vi "DoCreateError.vi"(5 "MergeErrors":bool, 6 "AdditionalText":string, 7 "Data":variant, 8 "ErrorIn":errorcluster caption="Error In", 9 "Text":string, 10 "ErrorCode":i32, 11 "ObjectIn":refnum<class "ErrorCreationJSON.lvclass"> caption="Object In") -> (0 "ErrorOut":errorcluster caption="Error Out", 3 "ObjectOut":refnum<class "ErrorCreationJSON.lvclass"> caption="Object Out")   [LabVIEW 2021, in "ErrorCreationJSON.lvclass"]
uses:
  ErrorCreationJSON.lvclass
  b793797b-a17e-43b8-8a57-7c74a2810d09.vi
  <vilib>/JDP Science/JSONtext/Variant to JSON Text.vi
  <vilib>/JDP Science/JSONtext/LVClass Serializer/JSONtext LVClass Serializer.lvclass
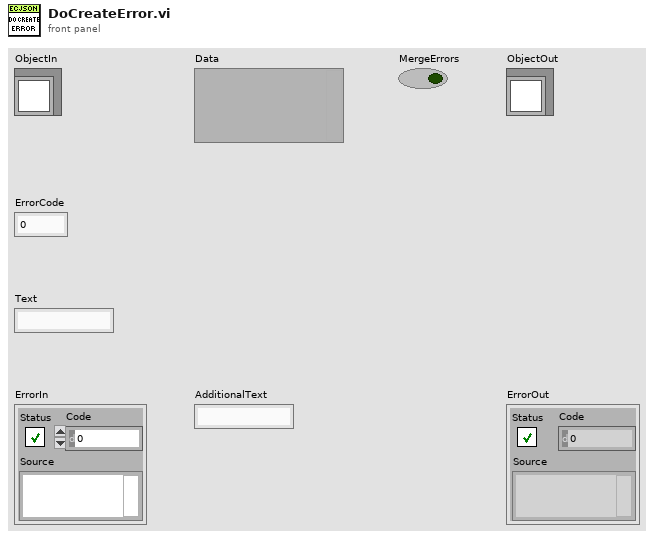
[diagram p1: front panel]
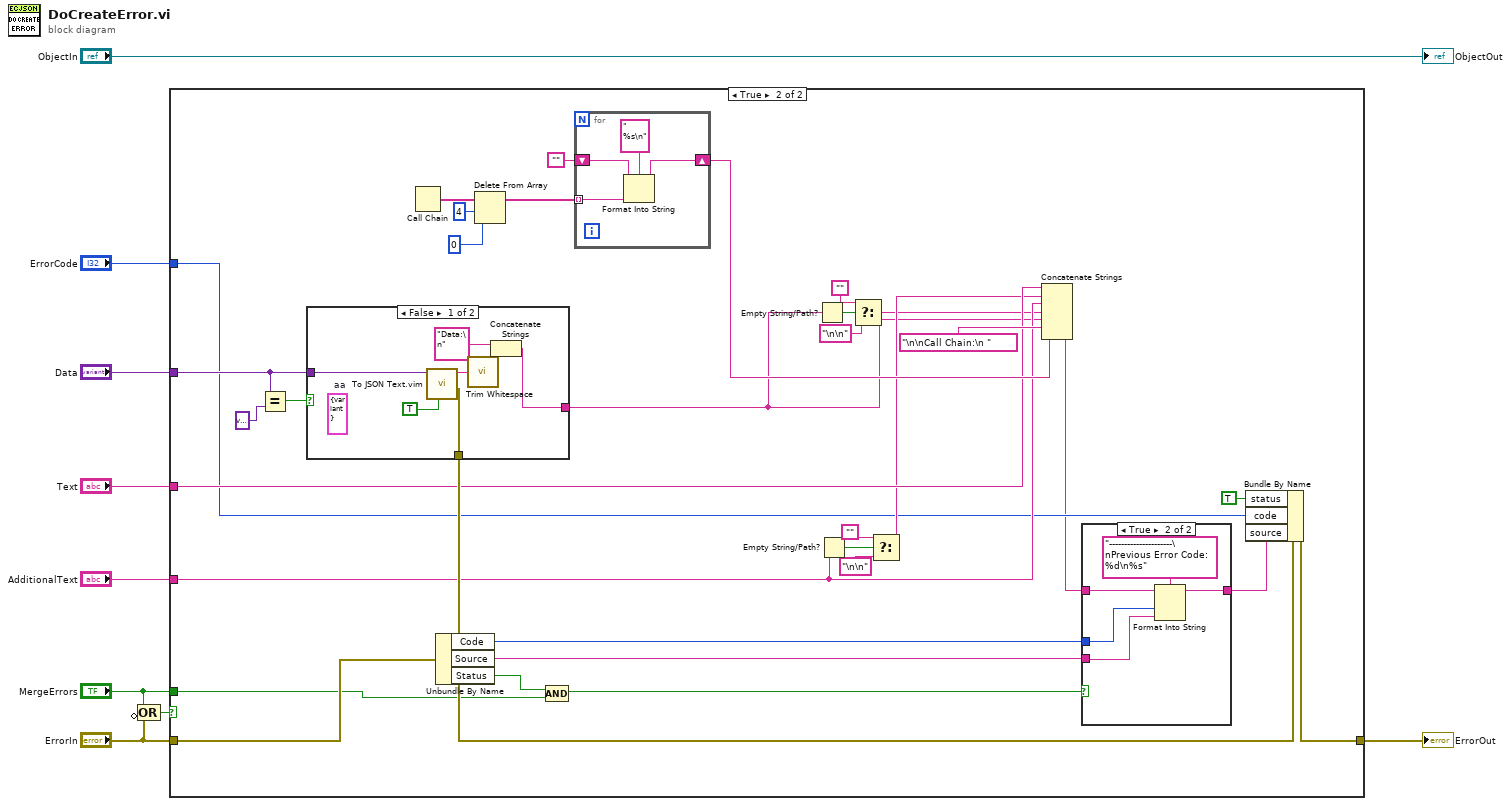
[diagram p0: block diagram]
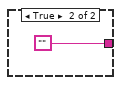
[diagram p4: hidden frame]
diagram:
  n1 = Compound Arithmetic op=OR("MergeErrors", invert "ErrorIn") -> (w2:bool)
  n2 = case shown="True" w2 {
    tunnel: "ErrorIn" -> [w10 w41]
    tunnel: [w10 w43] -> w9
    tunnel: "Data" -> [_ w40]
    tunnel: "Text" -> [_ w29]
    tunnel: "AdditionalText" -> [_ w23]
    tunnel: "ErrorCode" -> [_ w18]
    tunnel: "MergeErrors" -> [_ w17]
    frame False {
    }
    frame True {
      n3 = Equal?(x=w40, y=variant) -> (x = y?=w37:bool)
      n4 = case shown="False" w37 {
        tunnel: [w55 ""] -> w21
        tunnel: w40 -> [w56 _]
        tunnel: [w58 _] -> w42
        frame False {
          (unwired) cluster{"fff":variant} {"fff"=variant}  # aa
          n5 = call "To JSON Text.vim"("Pretty Print?"=TRUE, "Anything"=w56) -> ("error out"=w58:errorcluster, "<JSON>"=w59:string)  [unwired: 8 in]
          n6 = call <vilib>:"Trim Whitespace.vi"("string"=w59) -> ("trimmed string"=w60:string)  [unwired: 1 in]
          n7 = Concatenate Strings("Data:\n" ("string"), w60) -> (w55:string)
        }
        frame True {
        }
      }
      n8 = Call Chain() -> (call chain=w35:string[])
      n9 = Unbundle By Name(w41) -> ("Code"=w16:i32, "Source"=w15:string, "Status"=w11:bool)
      n10 = Delete From Array(array=w35, length=4, index=0 ("length")) -> (array with subset deleted=w34:string[])  [unwired: 1 out]
      n11 = Compound Arithmetic op=AND(w11, w17) -> (w12:bool)
      n12 = for {
        tunnel: w34 -> [w53] mode=indexing
        shift-right: [w51] -> w30
        shift-left: "" -> [w52]
        n13 = Format Into String(format string="  %s\n", initial string=w52, w53) -> (resulting string=w51:string)  [unwired: 1 in, 1 out]
      }
      n14 = Empty String/Path?(string/path=w21) -> (empty?=w25:bool)
      n15 = Empty String/Path?(string/path=w23) -> (empty?=w28:bool)
      n16 = Select(t="", s=w25, f="\n\n") -> (s? t:f=w22:string)
      n17 = Select(t="", s=w28, f="\n\n") -> (s? t:f=w24:string)
      n18 = Concatenate Strings(w29, w24, w23, w22, w21, "\n\nCall Chain:\n " ("format string"), w30) -> (w14:string)
      n19 = case shown="True" w12 {
        tunnel: w16 -> [_ w46]
        tunnel: w15 -> [_ w45]
        tunnel: w14 -> [w44 w49]
        tunnel: [w44 w48] -> w13
        frame False {
        }
        frame True {
          n20 = Format Into String(format string="---------------------\nPrevious Error Code: %d\n%s", initial string=w49, w46, w45) -> (resulting string=w48:string)  [unwired: 1 in, 1 out]
        }
      }
      n21 = Bundle By Name(cluster=w42, "status"=TRUE, "code"=w18, "source"=w13) -> (w43:errorcluster)
    }
  }
  "ErrorOut" <- w9
  "ObjectOut" <- "ObjectIn"
